vi "Set Source Item.vi"(7 "Source Index":i32, 8 "error in (no error)":errorcluster, 10 "Project Item":refnum<vi>, 11 "Build Spec in":refnum<vi>) -> (0 "error out":errorcluster, 3 "Build Spec out":refnum<vi>)   [LabVIEW 2019, in "Project Sync Tools.lvclass"]
uses:
  Project Sync Tools.lvclass
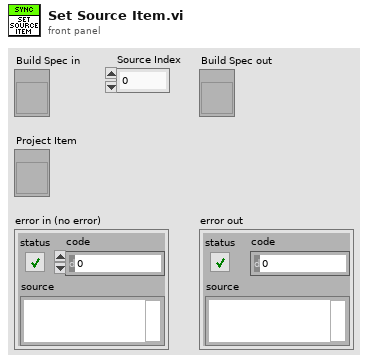
[diagram p1: front panel]
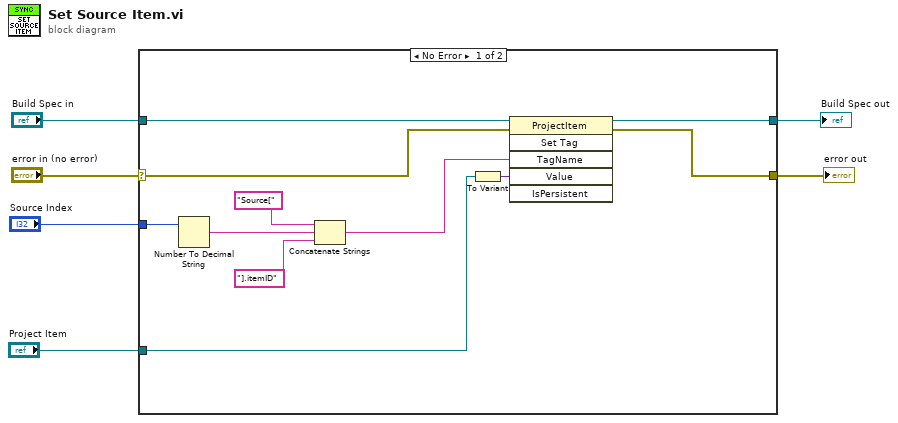
[diagram p0: block diagram]
diagram:
  n1 = case shown="No Error" "error in (no error)" {
    selector: "error in (no error)" -> [w7 w19]
    tunnel: "Project Item" -> [w16 _]
    tunnel: [w15 w19] -> w5
    tunnel: [w14 w18] -> w4
    tunnel: "Build Spec in" -> [w13 w18]
    tunnel: "Source Index" -> [w9 _]
    frame No Error {
      n2 = Number To Decimal String(number=w9) -> (decimal integer string=w11:string)  [unwired: 1 in]
      n3 = Concatenate Strings("Source[" ("string"), w11, "].itemID") -> (w8:string)
      n4 = To Variant(anything=w16) -> (Variant=w17:variant)
      n5 = invoke class="ProjectItem" method="Set Tag"(reference=w13, error in=w7, "TagName"=w8, "Value"=w17) -> (reference out=w14:refnum<vi>, error out=w15:errorcluster)  [unwired: 2 in, 4 out]
    }
    frame Error {
    }
  }
  "error out" <- w5
  "Build Spec out" <- w4
